vi "Get Value.vi"(8 "error in (no error)":errorcluster, 11 "Element A in":refnum<class "Element A.lvclass">) -> (0 "error out":errorcluster, 2 "Value":string, 3 "Element A out":refnum<class "Element A.lvclass">)   [LabVIEW 2020, in "Array Example.lvlib" / "Element A.lvclass"]
uses:
  Element A.lvclass
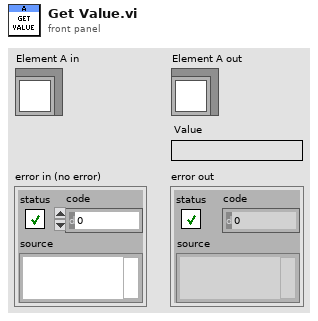
[diagram p1: front panel]
types:
  T1 = typedef "Array Example.lvlib/Element A.lvclass/Ref.ctl" = cluster{"Boolean":bool}
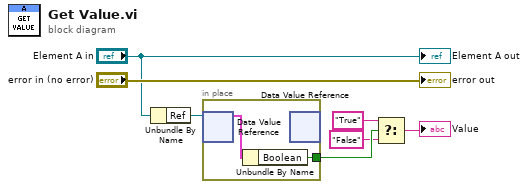
[diagram p0: block diagram]
diagram:
  n1 = Unbundle By Name("Element A in") -> ("Ref"=w6:refnum<data-value>)
  n2 = in-place {
    in-place-border: [w8] -> w4
    n3 = in-place-dvr #1(w6) -> (w9:T1)  [unwired: 1 out]
    n4 = Unbundle By Name(w9) -> ("Boolean"=w8:bool)
    n5 = in-place-dvr #1() -> ()  [unwired: 1 in, 2 out]
  }
  n6 = Select(t="True", s=w4, f="False") -> (s? t:f=→"Value":string)
  "error out" <- "error in (no error)"
  "Element A out" <- "Element A in"
